vi "WriteLogFile.vi"(5 "OK Button":bool, 6 "Automatic warning":string caption="Automatic warning (e.g. large Temperature/RH fluctuations)", 7 "Data File":string, 8 "Error In":errorcluster, 9 "DUT passed?":bool, 10 "Value TechSpec criteria":dbl, 11 "Files saved?":bool) -> (0 "Error Out":errorcluster)   [LabVIEW 2018]
uses:
  globals/QC_RunInformation.vi
panel:
  out "Cause for quitting measurement":string
  in  "Add comment":bool
  out "Type of measurement":string
  out "Logfile entry":string
  # "Write Logfile"
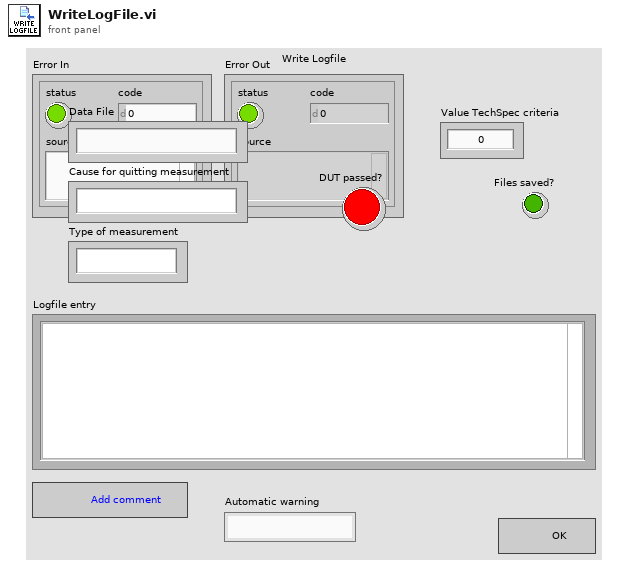
[diagram p1: front panel]
types:
  T1 = enum16{"open", "replace", "create", "open or create", "replace or create", "replace or create with confirmation"}
  T2 = cluster{"Sensor Serial No.:":string, "Wafer Serial No.:":string, "Batch:":string, "Manufacturer:":string, "Device Category:":string, "Database Serial No.:":string, "Date Initiated:":string, "Time Initiated:":string, "Test":string, "Instruments used:":string, "Probeplan used:":string, "End of Run comment:":string, "User:":string}
  T3 = cluster{"Institute":string, "Manufacturers":string[], "Devices":string[], "Serialnumbers Lookup DB":string, "Data directory":string, "Backup & screenshot directory":string, "List of known users":string[], "Measurement switch not used":bool, "Measurement Switch":string, "DUT Switch":string}
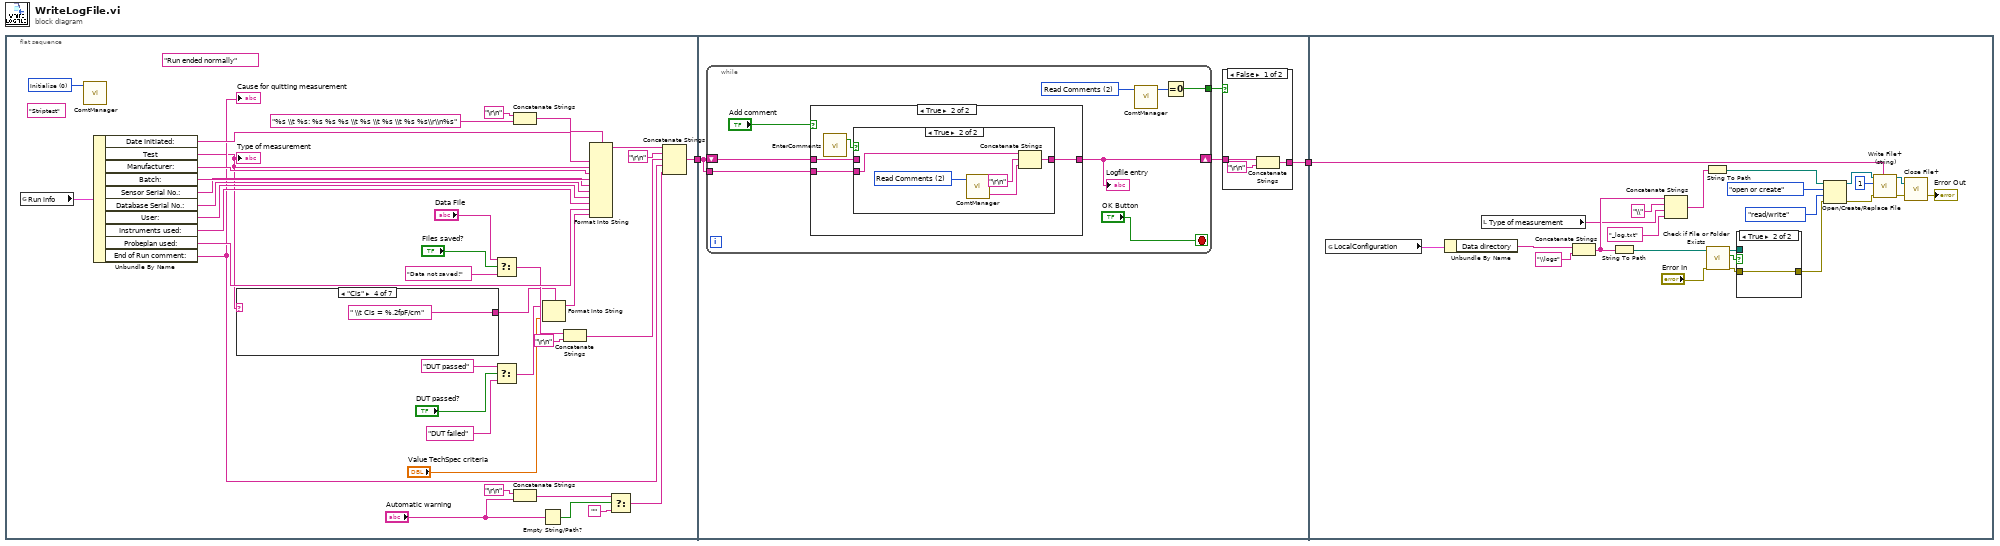
[diagram p0: block diagram]
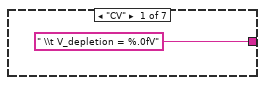
[diagram p2: hidden frame]
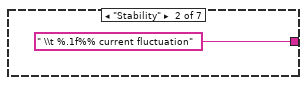
[diagram p3: hidden frame]
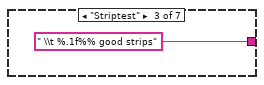
[diagram p4: hidden frame]
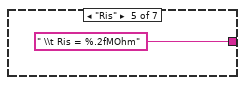
[diagram p5: hidden frame]
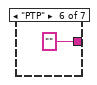
[diagram p6: hidden frame]
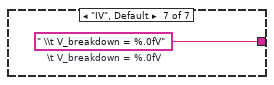
[diagram p7: hidden frame]
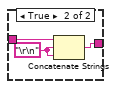
[diagram p8: hidden frame]
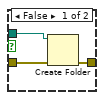
[diagram p11: hidden frame]
diagram:
  n1 = flat-sequence {
    tunnel: [w33] -> w2
    tunnel: w2 -> [w50]
    tunnel: [w48] -> w1
    tunnel: w1 -> [w91]
    frame #0 {
      (unwired) "Run ended normally" ("Cause for quitting measurement")
      (unwired) "Striptest"
      w32 = u16 0 items=["Initialise", "Add comment", "Read Comments"] ("Action")
      n2 = global read "QC_RunInformation.vi" "Run info"() -> (w31:T2)
      n3 = call "ComtManager.vi"("Action"=w32) -> ()  [unwired: 2 in, 3 out]
      n4 = Unbundle By Name(w31) -> ("Date Initiated:"=w39:string, "Test"=w12:string, "Manufacturer:"=w29:string, "Batch:"=w28:string, "Sensor Serial No.:"=w27:string, "Database Serial No.:"=w26:string, "User:"=w25:string, "Instruments used:"=w24:string, "Probeplan used:"=w23:string, "End of Run comment:"=w14:string)
      "Type of measurement" <- w12
      "Cause for quitting measurement" <- w14
      n5 = case shown="\"Cis\"" w12 {
        tunnel: [" \\t V_depletion = %.0fV" " \\t %.1f%% current fluctuation" " \\t %.1f%% good strips" " \\t Cis = %.2fpF/cm" " \\t Ris = %.2fMOhm" "" w46] -> w11
        frame "CV" {
        }
        frame "Stability" {
        }
        frame "Striptest" {
        }
        frame "Cis" {
        }
        frame "Ris" {
        }
        frame "PTP" {
        }
        frame "IV", Default {
          w46 = " \\t V_breakdown = %.0fV"  # \t V_breakdown = %.0fV
        }
      }
      n6 = Select(t="Data File", s="Files saved?", f="Data not saved!") -> (s? t:f=w16:string)
      n7 = Select(t="DUT passed", s="DUT passed?", f="DUT failed") -> (s? t:f=w10:string)
      n8 = Concatenate Strings("\r\n", "%s \\t %s: %s %s %s \\t %s \\t %s \\t %s %s\\r\\n%s") -> (w37:string)
      n9 = Concatenate Strings("\r\n", "Automatic warning") -> (w5:string)
      n10 = Empty String/Path?(string/path="Automatic warning") -> (empty?=w7:bool)
      n11 = Format Into String(format string=w11, initial string=w10, "Value TechSpec criteria") -> (resulting string=w9:string)  [unwired: 1 in, 1 out]
      n12 = Concatenate Strings(w16, "\r\n") -> (w34:string)
      n13 = Format Into String(format string=w37, w39, w12, w29, w28, w27, w26, w25, w24, w23, w9) -> (resulting string=w35:string)  [unwired: 2 in, 1 out]
      n14 = Select(t=w5, s=w7, f="") -> (s? t:f=w3:string)
      n15 = Concatenate Strings(w35, "\r\n", w34, w14, w3) -> (w33:string)
    }
    frame #1 {
      n16 = while {
        shift-right: [w61] -> w49
        shift-left: w50 -> [w63]
        tunnel: w50 -> [w62]
        tunnel: [w58] -> w47
        stop <- "OK Button" stop-if-true
        w60 = u16 2 items=["Initialise", "Add comment", "Read Comments"] ("Action")
        n17 = case shown="True" "Add comment" {
          tunnel: [w65 w68] -> w61
          tunnel: w63 -> [w65 w67]
          tunnel: w62 -> [_ w66]
          frame False {
          }
          frame True {
            n18 = call "EnterComments.vi"() -> ("update?"=w69:bool)  [unwired: 4 in]
            n19 = case shown="True" w69 {
              tunnel: [w70 w74] -> w68
              tunnel: w67 -> [w70 _]
              tunnel: w66 -> [_ w73]
              frame False {
              }
              frame True {
                w75 = u16 2 items=["Initialise", "Add comment", "Read Comments"] ("Action")
                n20 = call "ComtManager.vi"("Action"=w75) -> ("Comment out"=w72:string)  [unwired: 2 in, 2 out]
                n21 = Concatenate Strings(w73, "\r\n", w72) -> (w74:string)
              }
            }
          }
        }
        "Logfile entry" <- w61
        n22 = call "ComtManager.vi"("Action"=w60) -> ("No of comments"=w59:i32)  [unwired: 2 in, 2 out]
        n23 = Equal To 0?(x=w59) -> (x = 0?=w58:bool)
      }
      n24 = case shown="False" w47 {
        tunnel: w49 -> [w52 w54]
        tunnel: [w51 w55] -> w48
        frame False {
          n25 = Concatenate Strings(w52, "\r\n") -> (w51:string)
        }
        frame True {
          w56 = "\r\n"
          n26 = Concatenate Strings(w54, w56, w56) -> (w55:string)
        }
      }
    }
    frame #2 {
      n27 = global read "QC_RunInformation.vi" "LocalConfiguration"() -> (w90:T3)
      n28 = Unbundle By Name(w90) -> ("Data directory"=w88:string)
      n29 = local read "Type of measurement"() -> (w76:string)
      n30 = Concatenate Strings(w88, "\\logs") -> (w85:string)
      n31 = String To Path(string=w85) -> (path=w82:path)
      n32 = Concatenate Strings(w85, "\\", w76, "_log.txt") -> (w84:string)
      n33 = String To Path(string=w84) -> (path=w83:path)
      n34 = call <vilib>:"Check if File or Folder Exists.vi"("error in (no error)"="Error In", "path"=w82) -> ("error out"=w78:errorcluster, "file or folder exists?"=w81:bool, "dup path"=w80:path)  [unwired: 7 in]
      n35 = case shown="True" w81 {
        tunnel: w80 -> [w102 _]
        tunnel: w78 -> [w101 w103]
        tunnel: [w100 w103] -> w77
        frame False {
          n36 = Create Folder(path (use dialog)=w102, error in=w101) -> (error out=w100:errorcluster)  [unwired: 1 in, 2 out]
        }
        frame True {
        }
      }
      n37 = Open/Create/Replace File(file path (use dialog)=w83, error in=w77, operation (0:open)=T1."open or create", access (0:read/write)=enum16{"read/write", "read-only", "write-only"}."read/write") -> (refnum out=w96:refnum<file>, error out=w97:errorcluster)  [unwired: 2 in, 1 out]
      n38 = call <vilib>:"Write File+ (string).vi"("string"=w91, "error in (no error)"=w97, "pos mode (rel. to end:1)"=1, "refnum"=w96) -> ("error out"=w93:errorcluster, "dup refnum"=w92:refnum<file>)  [unwired: 3 in, 1 out]
      n39 = call <vilib>:"Close File+.vi"("error in (no error)"=w93, "refnum"=w92) -> ("error out"=→"Error Out":errorcluster)  [unwired: 3 in, 2 out]
    }
  }
